vi "test Multiple Clients - WebSockets Secure.vi"(8 "error in (no error)":errorcluster, 11 "TestCase in":refnum<class "test Multiple Clients.lvclass">) -> (0 "error out":errorcluster, 3 "TestCase out":refnum<class "test Multiple Clients.lvclass">)   [LabVIEW 2013, in "test Multiple Clients.lvclass"]
uses:
  test Multiple Clients.lvclass
  dotNET SSL Socket/dotNET WebSocket/Server/Server SSL Options.ctl
  dotNET SSL Socket/dotNET SSL Socket/PFX Certificate.ctl
  dotNET SSL Socket/dotNET SSL Listener/dotNET Listener.lvclass
  dotNET SSL Socket/dotNET WebSocket/Server/dotNET WebSocket Server.lvclass
  dotNET SSL Socket/dotNET WebSocket/Client/dotNET WebSocket Client.lvclass
  <vilib>/addons/_JKI Toolkits/VI Tester/TestCase.llb/TestCase.lvclass
  dotNET SSL Socket/dotNET SSL Socket/dotNET SSL Socket.lvclass
panel:
  out "Client Received":i32[](array[numeric])
  out "Server Received Length":i32[](array[numeric])
  out "Sent Length":i32[](array[numeric])
  out "x = y?":bool
  out "Sent":string[](array[string])
  out "Received by Server":string[](array[string])
  out "Returned":string[](array[string])
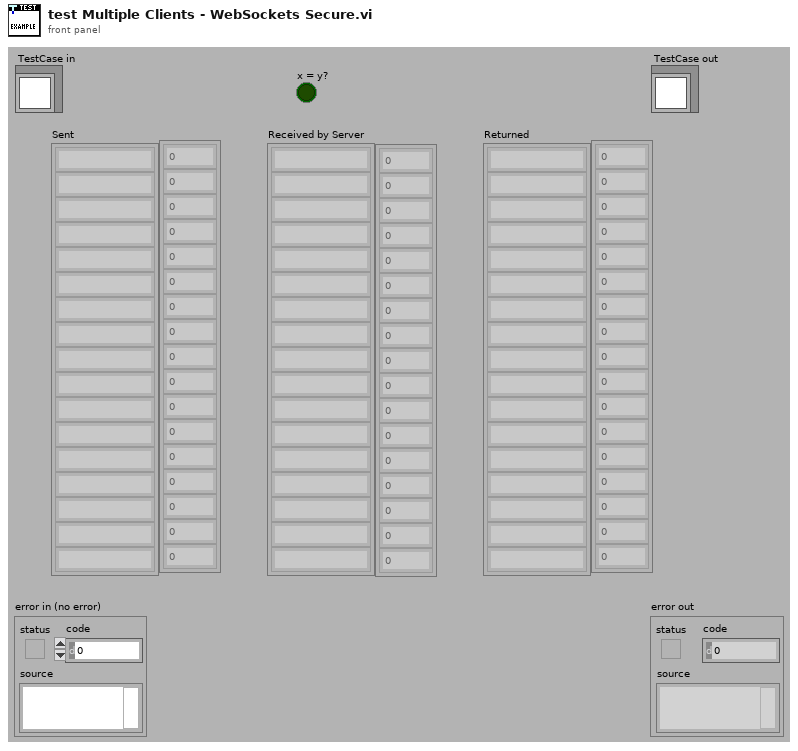
[diagram p1: front panel]
types:
  T1 = typedef "dotNET WebSocket.lvlib/dotNET WebSocket Server.lvclass/Server SSL Options.ctl" = cluster{"Check Revocation":bool, "Client Cert Required":bool, "Server Certificate":T2, "SSL Protocols":i32[]}
  T2 = typedef "dotNET SSL Socket.lvlib/dotNET SSL Socket.lvclass/PFX Certificate.ctl" = cluster{"PFX Certificate":path, "PFX Password":string}
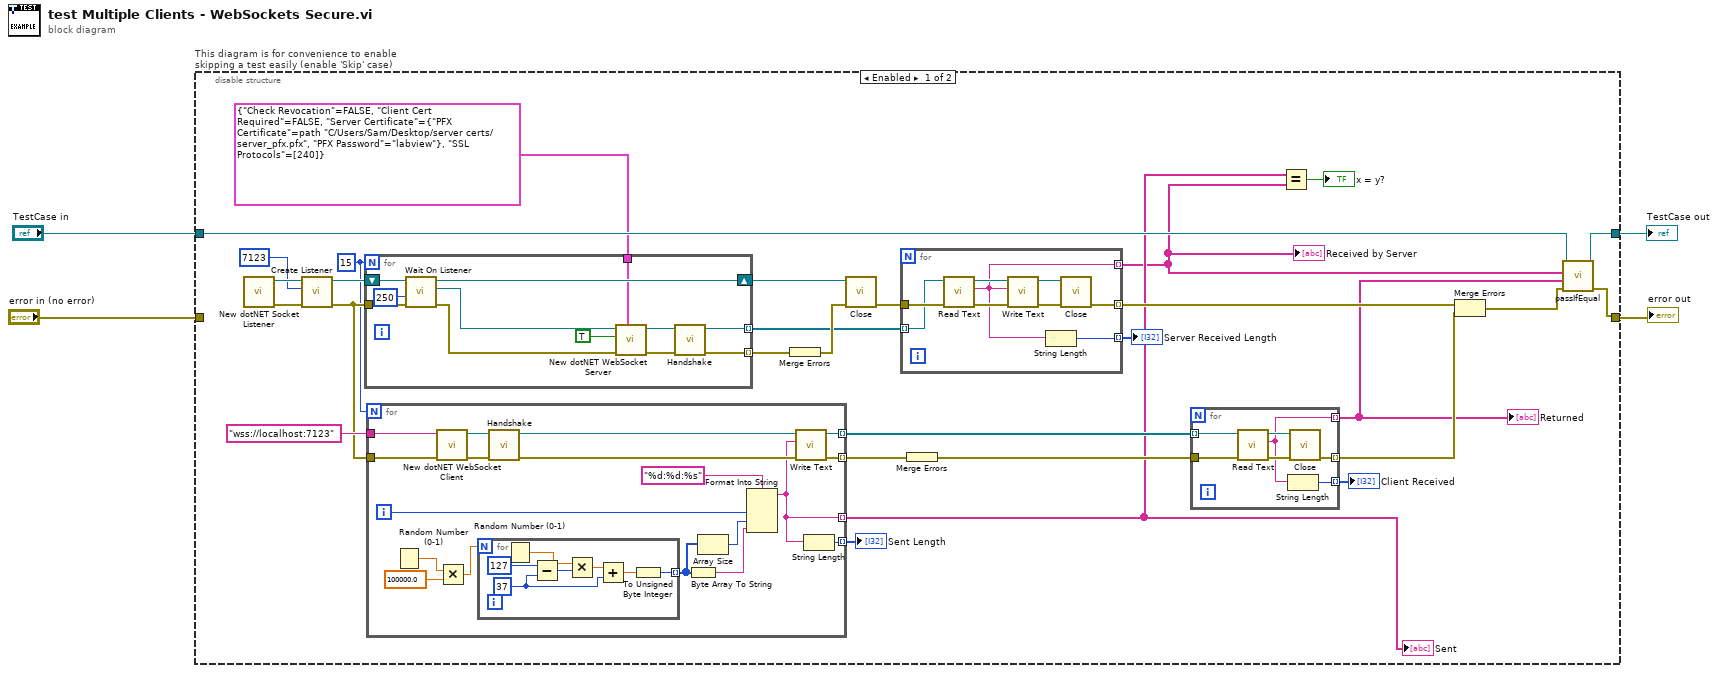
[diagram p0: block diagram]
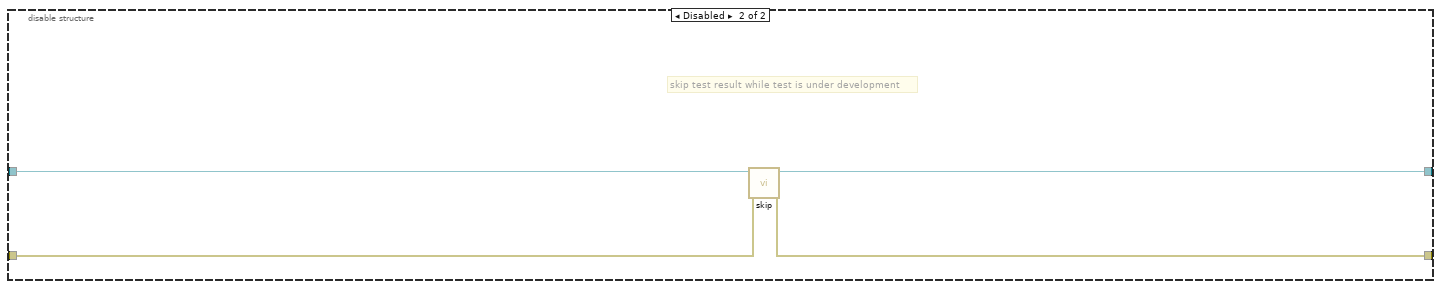
[diagram p2: hidden frame]
diagram:
  n1 = disable-structure "This diagram is for convenience to enable skipping a test easily (enable 'Skip' case)" shown="Enabled" {
    disable-tunnel: "TestCase in" -> [w33 w90]
    disable-tunnel: [w32 w88] -> w1
    disable-tunnel: [w31 w89] -> w3
    disable-tunnel: "error in (no error)" -> [_ w87]
    frame Enabled {
      w19 = 15
      n2 = call "New dotNET Socket Listener.vi"() -> ("error out"=w30:errorcluster, "dotNET Listener out"=w29:refnum<class "dotNET Listener.lvclass">)  [unwired: 10 in]
      n3 = call-dynamic "Create Listener.vi"("error in (no error)"=w30, "Port"=u16 7123, "dotNET Listener in"=w29) -> ("error out"=w25:errorcluster, "dotNET Listener out"=w28:refnum<class "dotNET Listener.lvclass">)  [unwired: 7 in]
      n4 = for {
        N: w19 -> [_]
        tunnel: w25 -> [w85]
        shift-right: [w84] -> w23
        shift-left: w28 -> [w86]
        tunnel: [w77] -> w24 mode=indexing
        tunnel: [w76] -> w21 mode=indexing
        tunnel: T1 {"Check Revocation"=FALSE, "Client Cert Required"=FALSE, "Server Certificate"={"PFX Certificate"=path "C:/Users/Sam/Desktop/server certs/server_pfx.pfx", "PFX Password"="labview"}, "SSL Protocols"=[240]} ("Server SSL Options (wss://)") -> [w80]
        n5 = call-dynamic "Wait On Listener.vi"("error in (no error)"=w85, "timeout ms (5000)"=250, "dotNET Listener in"=w86) -> ("error out"=w81:errorcluster, "Socket out"=w82:refnum<class "Socket.lvclass">, "dotNET Listener out"=w84:refnum<class "dotNET Listener.lvclass">)  [unwired: 6 in]
        n6 = call "New dotNET WebSocket Server.vi"("Server SSL Options (wss://)"=w80, "error in (no error)"=w81, "Use SSL?"=TRUE, "Socket in"=w82) -> ("error out"=w78:errorcluster, "dotNET WebSocket Server out"=w79:refnum<class "dotNET WebSocket Server.lvclass">)  [unwired: 6 in]
        n7 = call-dynamic "Handshake.vi"("error in (no error)"=w78, "WebSocket Connection in"=w79) -> ("error out"=w77:errorcluster, "WebSocket Connection out"=w76:refnum<class "dotNET WebSocket Server.lvclass">)  [unwired: 8 in]
      }
      n8 = for {
        N: w19 -> [_]
        tunnel: "wss://localhost:7123" ("Hostname / URL") -> [w61]
        tunnel: w25 -> [w62]
        tunnel: [w51] -> w10 mode=indexing
        tunnel: [w65] -> w17 mode=indexing
        tunnel: [w64] -> w16 mode=indexing
        tunnel: [w50] -> w7 mode=indexing
        i -> [w67]
        n9 = Random Number (0-1)() -> (number: 0 to 1=w57:dbl)
        n10 = call "New dotNET WebSocket Client.vi"("error in (no error)"=w62, "WebSocket URL"=w61) -> ("error out"=w63:errorcluster, "dotNET WS Client out"=w60:refnum<class "dotNET WebSocket Client.lvclass">)  [unwired: 8 in]
        n11 = Multiply(x=w57, y=100000.0) -> (x*y=w55:dbl)
        n12 = for {
          N: w55 -> [_]
          tunnel: [w68] -> w54 mode=indexing
          w70 = u8 37 ("lower limit")
          n13 = Random Number (0-1)() -> (number: 0 to 1=w72:dbl)
          n14 = Subtract(x=u8 127 ("upper limit"), y=w70) -> (x-y=w71:u8)
          n15 = Multiply(x=w72, y=w71) -> (x*y=w73:dbl)
          n16 = Add(x=w73, y=w70) -> (x+y=w69:dbl)
          n17 = To Unsigned Byte Integer(number=w69) -> (unsigned 8bit integer=w68:u8)
        }
        n18 = call-dynamic "Handshake.vi"("error in (no error)"=w63, "WebSocket Client in"=w60) -> ("error out"=w58:errorcluster, "WebSocket Client out"=w59:refnum<class "dotNET WebSocket Client.lvclass">)  [unwired: 8 in]
        n19 = Byte Array To String(unsigned byte array=w54) -> (string=w52:string)
        n20 = Array Size(array=w54) -> (size(s)=w53:i32)
        n21 = Format Into String(format string="%d:%d:%s", w67, w53, w52) -> (resulting string=w51:string)  [unwired: 2 in, 1 out]
        n22 = call-dynamic "Write Text.vi"("error in (no error)"=w58, "String Data"=w51, "WebSocket in"=w59) -> ("error out"=w64:errorcluster, "WebSocket out"=w65:refnum<class "dotNET WebSocket Client.lvclass">)  [unwired: 7 in]
        n23 = String Length(string=w51) -> (length=w50:i32)
      }
      "Sent" <- w10
      "Sent Length" <- w7
      n24 = Merge Errors(w24) -> (w22:errorcluster)
      n25 = call-dynamic "Close.vi"("error in (no error)"=w22, "dotNET Listener in"=w23) -> ("error out"=w20:errorcluster)  [unwired: 9 in]
      n26 = for {
        tunnel: w21 -> [w48] mode=indexing
        tunnel: w20 -> [w49]
        tunnel: [w42] -> w9 mode=indexing
        tunnel: [w43] -> w18 mode=indexing
        tunnel: [w41] -> w6 mode=indexing
        n27 = call-dynamic "Read Text.vi"("error in (no error)"=w49, "WebSocket in"=w48) -> ("error out"=w46:errorcluster, "Data"=w42:string, "WebSocket out"=w47:refnum<class "dotNET WebSocket Server.lvclass">)  [unwired: 7 in]
        n28 = call-dynamic "Write Text.vi"("error in (no error)"=w46, "String Data"=w42, "WebSocket in"=w47) -> ("error out"=w45:errorcluster, "WebSocket out"=w44:refnum<class "dotNET WebSocket Server.lvclass">)  [unwired: 7 in]
        n29 = String Length(string=w42) -> (length=w41:i32)
        n30 = call-dynamic "Close.vi"("error in (no error)"=w45, "WebSocket in"=w44) -> ("error out"=w43:errorcluster)  [unwired: 9 in]
      }
      "Received by Server" <- w9
      "Server Received Length" <- w6
      n31 = Merge Errors(w16) -> (w15:errorcluster)
      n32 = for {
        tunnel: w17 -> [w40] mode=indexing
        tunnel: w15 -> [w39]
        tunnel: [w36] -> w14 mode=indexing
        tunnel: [w35] -> w11 mode=indexing
        tunnel: [w34] -> w5 mode=indexing
        n33 = call-dynamic "Read Text.vi"("error in (no error)"=w39, "WebSocket in"=w40) -> ("error out"=w38:errorcluster, "Data"=w35:string, "WebSocket out"=w37:refnum<class "dotNET WebSocket Client.lvclass">)  [unwired: 7 in]
        n34 = String Length(string=w35) -> (length=w34:i32)
        n35 = call-dynamic "Close.vi"("error in (no error)"=w38, "WebSocket in"=w37) -> ("error out"=w36:errorcluster)  [unwired: 9 in]
      }
      "Returned" <- w11
      "Client Received" <- w5
      n36 = Equal?(x=w10, y=w9) -> (x = y?=→"x = y?":bool)
      n37 = Merge Errors(w18, w14) -> (w13:errorcluster)
      n38 = call-dynamic "passIfEqual.vi"("error in (no error)"=w13, "y"=w11, "x"=w9, "TestCase in"=w33) -> ("error out"=w31:errorcluster, "TestCase out"=w32:refnum<class "test Multiple Clients.lvclass">)  [unwired: 6 in]
    }
    frame Disabled {
      # "skip test result while test is under development"
      n39 = call <vilib>:"skip.vi"("error in (no error)"=w87, "TestCase in"=w90) -> ("error out"=w89:errorcluster, "TestCase out"=w88:refnum<class "test Multiple Clients.lvclass">)  [unwired: 8 in]
    }
  }
  "error out" <- w3
  "TestCase out" <- w1
